vi "vipmGetInstalled.vi"   [LabVIEW 2017, in "vipm-build-tools.lvlib"]
uses:
  vipm-build-tools.lvlib
  <vilib>/JKI/VIPM API/VIPM API_vipm_api.lvlib
  <vilib>/Wiresmith Technology/LabVIEW CLI/CLI Class/CLI.lvclass
types:
  T1 = enum16{"open", "replace", "create", "open or create", "replace or create", "replace or create with confirmation"}
  T2 = typedef "VIPM API_vipm_api.lvlib/Library Contents Cluster_vipm_api.ctl" = cluster{"Package Name":string, "Version":string, "Display Name":string, "Repository Name":string, "Company Name":string, "License Type":string, "Installed":bool, "Deprecated":bool, "Dependency or Conflict Problem":bool, "Downloaded":bool}
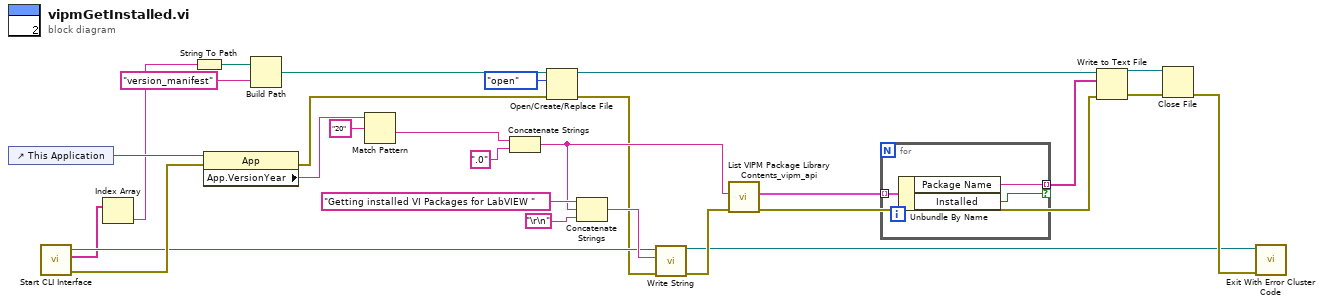
[diagram p0: block diagram]
diagram:
  n1 = control-ref of="This Application"() -> (w28:refnum<vi>)
  n2 = call <vilib>:"Start CLI Interface.vi"() -> ("error out"=w23:errorcluster, "Custom Parameters"=w16:string[], "CLI out"=w17:refnum<class "CLI.lvclass">)  [unwired: 9 in]
  n3 = Index Array(array=w16) -> (element=w15:string)  [unwired: 1 in]
  n4 = String To Path(string=w15) -> (path=w14:path)
  n5 = property class="App"(reference=w28, error in=w23) -> (error out=w11:errorcluster, "App.VersionYear"=w27:string)  [unwired: 1 out]
  n6 = Build Path(base path=w14, name or relative path="version_manifest") -> (appended path=w12:path)
  n7 = Match Pattern(string=w27, regular expression="20") -> (after substring=w24:string)  [unwired: 1 in, 3 out]
  n8 = Concatenate Strings(w24, ".0" ("format string")) -> (w18:string)
  n9 = Open/Create/Replace File(file path (use dialog)=w12, error in=w11, operation (0:open)=T1."open") -> (refnum out=w5:refnum<file>, error out=w10:errorcluster)  [unwired: 3 in, 1 out]
  n10 = Concatenate Strings("Getting installed VI Packages for LabVIEW " ("Text to Write"), w18, "\r\n") -> (w22:string)
  n11 = call <vilib>:"Write String.vi"("error in (no error)"=w10, "Text to Write"=w22, "CLI in"=w17) -> ("error out"=w19:errorcluster, "CLI out"=w1:refnum<class "CLI.lvclass">)  [unwired: 7 in]
  n12 = call <vilib>:"List VIPM Package Library Contents_vipm_api.vi"("error in (no error)"=w19, "LabVIEW Version"=w18) -> ("error out"=w7:errorcluster, "Library Contents []"=w8:T2[])  [unwired: 8 in]
  n13 = for {
    tunnel: w8 -> [w31] mode=indexing
    tunnel: [w30] -> w6 mode=indexing if=w29
    n14 = Unbundle By Name(w31) -> ("Package Name"=w30:string, "Installed"=w29:bool)
  }
  n15 = Write to Text File(file (use dialog)=w5, text=w6, error in=w7) -> (refnum out=w3:refnum<file>, error out=w4:errorcluster)  [unwired: 1 in, 1 out]
  n16 = Close File(refnum=w3, error in=w4) -> (error out=w2:errorcluster)  [unwired: 1 out]
  n17 = call <vilib>:"Exit With Error Cluster Code.vi"("error in (no error)"=w2, "CLI in"=w1) -> ()  [unwired: 9 in, 1 out]
